vi "DB5000.R写.vi"(0 "gInitialSIEMENSS7 In":refnum<k24>, 1 "地址数组":string[](array[string])=["DB5000.136", "DB5000.140", "DB5000.144", "DB5000.148", "DB5000.152", "DB5000.156", "DB5000.160", "DB5000.164", "DB5000.168", "DB5000.172", "DB5000.176"], 5 "error in (no error)":errorcluster caption="错误输入（无错误）") -> (14 "gInitialSIEMENSS7 Out":refnum<k24>, 15 "IsSuccess":bool, 17 "添加的数组":sgl[](array[numeric]), 19 "error out":errorcluster caption="错误输出")   [LabVIEW 2017]
panel:
  # "DB5000,REAL136"
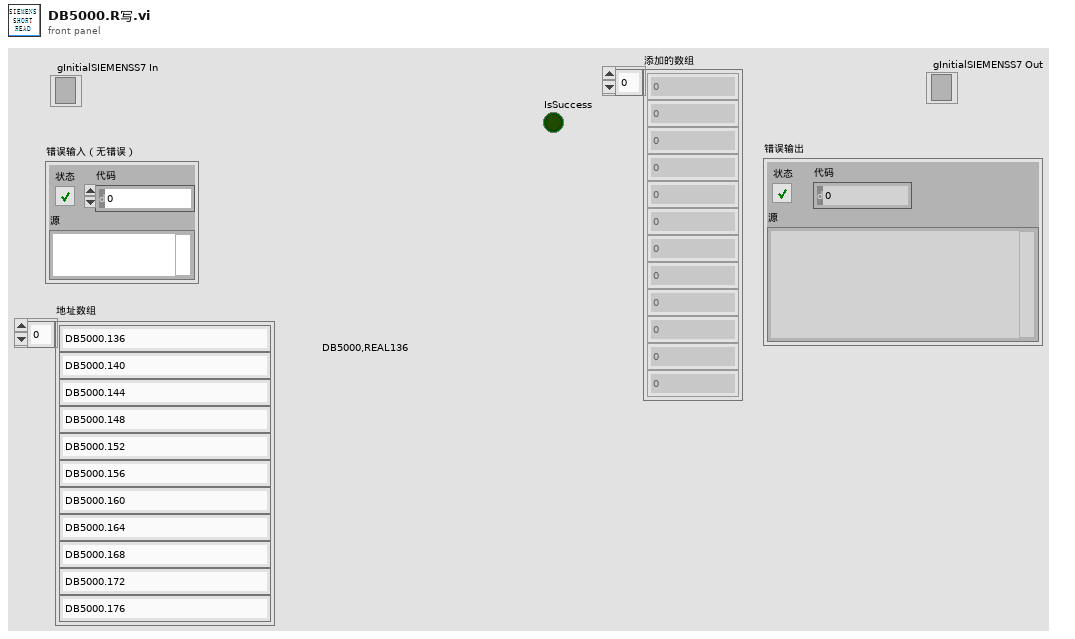
[diagram p1: front panel]
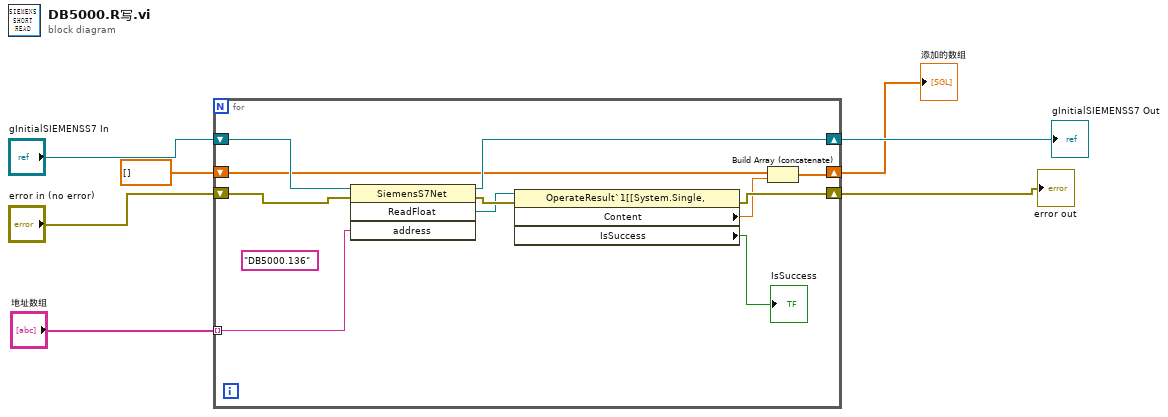
[diagram p0: block diagram]
diagram:
  n1 = for {
    shift-right: [w13] -> w4
    shift-left: "gInitialSIEMENSS7 In" -> [w18]
    shift-right: [w14] -> w5
    shift-left: "error in (no error)" -> [w17]
    tunnel: "地址数组" -> [w12] mode=indexing
    shift-right: [w9] -> w1
    shift-left: sgl[] [] ("添加的数组") -> [w10]
    (unwired) "DB5000.136" ("address")
    n2 = invoke class="SiemensS7Net" method="ReadFloat"(reference=w18, error in=w17, "address"=w12) -> (reference out=w13:refnum<k24>, error out=w16:errorcluster, "ReadFloat"=w15:refnum<k24>)  [unwired: 1 in, 1 out]
    n3 = property class="OperateResult`1[[System.Single,"(reference=w15, error in=w16) -> (error out=w14:errorcluster, "Content"=w11:sgl, "IsSuccess"=→"IsSuccess":bool)  [unwired: 1 out]
    n4 = Build Array (concatenate)(w10, w11) -> (w9:sgl[])
  }
  "gInitialSIEMENSS7 Out" <- w4
  "error out" <- w5
  "添加的数组" <- w1
